vi "Get Library Key with Raw Name Cacher.vi"(10 "key":string) -> (1 "Raw name":string, 2 "Key in lower case":string, 6 "cacher":variant)   [LabVIEW 2017]
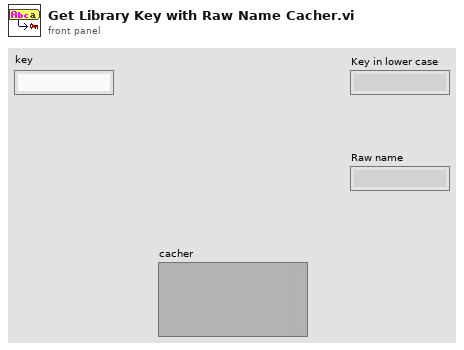
[diagram p1: front panel]
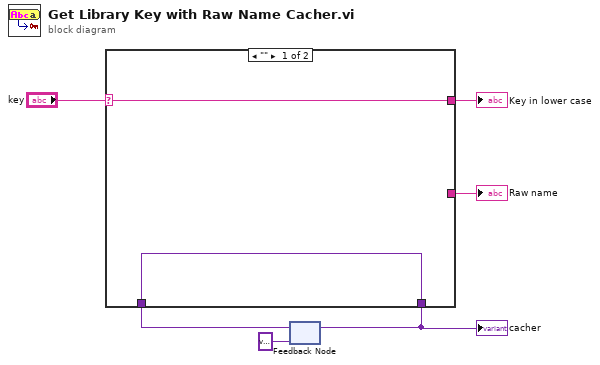
[diagram p0: block diagram]
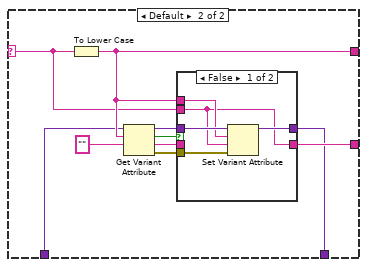
[diagram p2: hidden frame]
diagram:
  n1 = feedback #1(variant) -> (w2:variant)
  n2 = case shown="\"\"" "key" {
    selector: "key" -> [w8 w14]
    tunnel: [w8 w17] -> w6
    tunnel: [_ w11] -> w4
    tunnel: w2 -> [w7 w10]
    tunnel: [w7 w9] -> w1
    frame "" {
    }
    frame Default {
      n3 = To Lower Case(string=w14) -> (all lower case string=w17:string)
      n4 = Get Variant Attribute(Variant=w10, name=w17, default value (empty Variant)="") -> (duplicate Variant=w18:variant, found=w15:bool, value=w13:string, error out=w12:errorcluster)  [unwired: 1 in]
      n5 = case shown="False" w15 {
        tunnel: w18 -> [w23 w25]
        tunnel: w17 -> [w22 _]
        tunnel: w14 -> [w19 _]
        tunnel: w13 -> [_ w24]
        tunnel: w12 -> [w21 _]
        tunnel: [w20 w25] -> w9
        tunnel: [w19 w24] -> w11
        frame False {
          n6 = Set Variant Attribute(Variant=w23, name=w22, value=w19, error in=w21) -> (Variant out=w20:variant)  [unwired: 2 out]
        }
        frame True {
        }
      }
    }
  }
  "Key in lower case" <- w6
  "Raw name" <- w4
  "cacher" <- w1
  n7 = feedback-in #1(w1) -> ()
